vi "范围内渐变-颜色.vi"() -> ()   [LabVIEW 2013]
panel:
  in  "呼吸间隔ms":u32=250
  in  "刷新频率ms":u32=20
  out "波形图表":dbl(graph)
  out "Color":u32(colorbox) caption="颜色"
  in  "B动态范围":u8(slide) scale=1.0..50.0
  in  "R常量":u8(slide) scale=0.0..255.0
  in  "停止按钮":bool
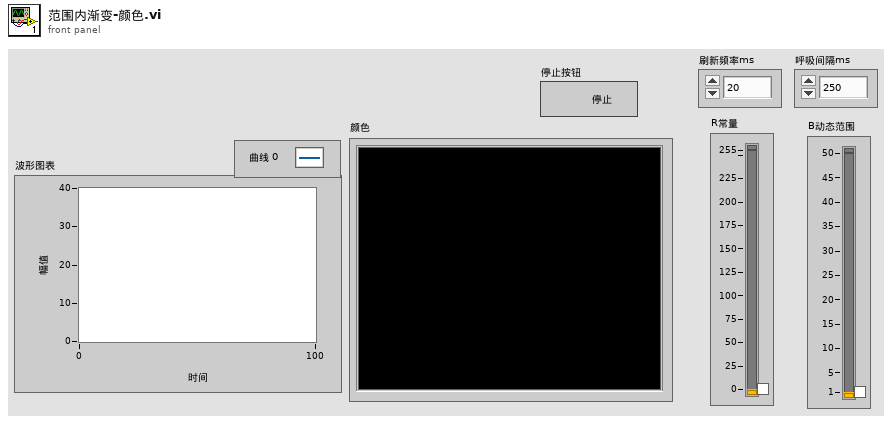
[diagram p1: front panel]
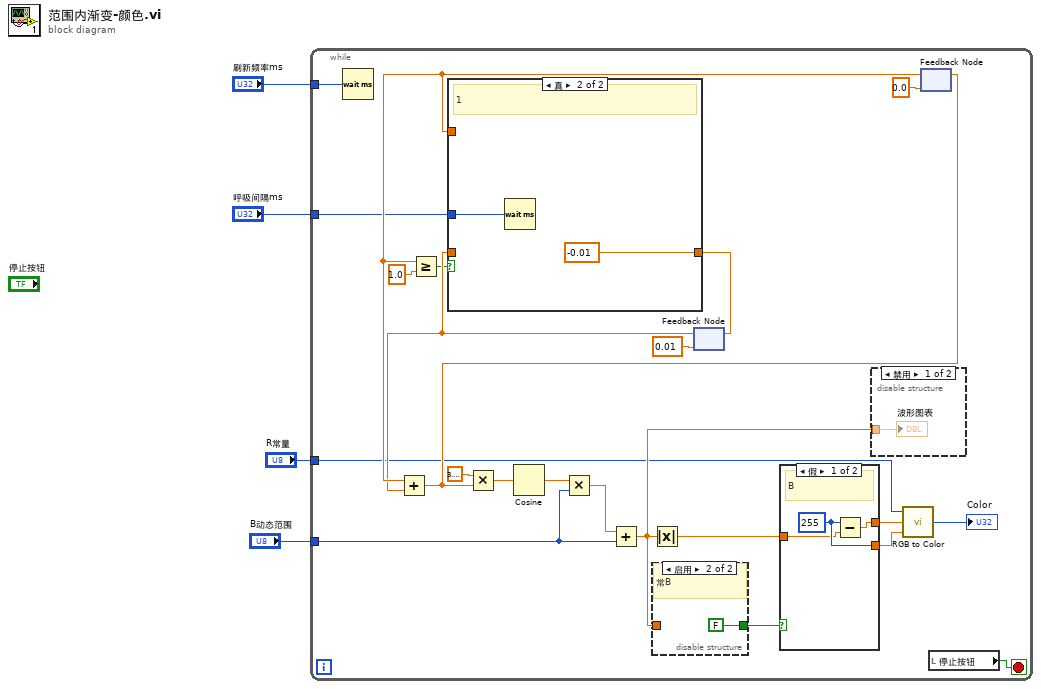
[diagram p0: block diagram]
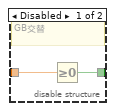
[diagram p3: hidden frame]
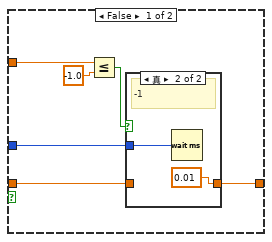
[diagram p4: hidden frame]
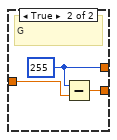
[diagram p6: hidden frame]
diagram:
  n1 = while {
    tunnel: "刷新频率ms" -> [w8]
    tunnel: "呼吸间隔ms" -> [w7]
    tunnel: "B动态范围" -> [w6]
    tunnel: "R常量" -> [w5]
    stop <- w22 stop-if-true
    n2 = Wait (ms)(milliseconds to wait=w8) -> ()  [unwired: 1 out]
    n3 = feedback #1(0.01 ("y")) -> (w13:dbl)
    n4 = feedback #2(0.0 ("y")) -> (w15:dbl)
    n5 = Add(x=w15, y=w13) -> (x+y=w18:dbl)
    n6 = Greater Or Equal?(x=w15, y=1.0) -> (x >= y?=w10:bool)
    n7 = case shown="真" w10 {
      tunnel: [w34 -0.01 ("y")] -> w12
      tunnel: w15 -> [w37 _]
      tunnel: w13 -> [w35 _]
      tunnel: w7 -> [w32 w41]
      frame False {
        n8 = Less Or Equal?(x=w37, y=-1.0) -> (x <= y?=w33:bool)
        n9 = case shown="真" w33 {
          tunnel: w35 -> [w38 _]
          tunnel: [w38 0.01 ("y")] -> w34
          tunnel: w32 -> [_ w39]
          frame False {
          }
          frame True {
            # "-1"
            n10 = Wait (ms)(milliseconds to wait=w39) -> ()  [unwired: 1 out]
          }
        }
      }
      frame True {
        # "1"
        n11 = Wait (ms)(milliseconds to wait=w41) -> ()  [unwired: 1 out]
      }
    }
    n12 = Multiply(x=3.141592653589793, y=w18) -> (x*y=w20:dbl)
    n13 = Cosine(x=w20) -> (cos(x)=w21:dbl)
    n14 = Multiply(x=w21, y=w6) -> (x*y=w11:dbl)
    n15 = Add(x=w11, y=w6) -> (x+y=w9:dbl)
    n16 = Absolute Value(x=w9) -> (abs(x)=w23:dbl)
    n17 = disable-structure shown="启用" {
      disable-tunnel: [w30 FALSE] -> w26
      disable-tunnel: w9 -> [w29 _]
      frame Disabled {
        # "GB交替"
        n18 = Greater Or Equal To 0?(x=w29) -> (x >= 0?=w30:bool)
      }
      frame Enabled {
        # "常B"
      }
    }
    n19 = feedback-in #1(w12) -> ()
    n20 = case shown="假" w26 {
      tunnel: w23 -> [w44 w48]
      tunnel: [w45 w47] -> w25
      tunnel: [w43 w46] -> w24
      frame False {
        w45 = u8 255 ("G")
        # "B"
        n21 = Subtract(x=w45, y=w44) -> (x-y=w43:dbl)
      }
      frame True {
        w46 = u8 255 ("G")
        # "G"
        n22 = Subtract(x=w46, y=w48) -> (x-y=w47:dbl)
      }
    }
    n23 = disable-structure shown="禁用" {
      disable-tunnel: w9 -> [w28 _]
      frame Disabled {
        "波形图表" <- w28
      }
      frame Enabled {
      }
    }
    n24 = call <vilib>:"RGB to Color.vi"("B"=w25, "G"=w24, "R"=w5) -> ("Color"=→"Color":u32)
    n25 = feedback-in #2(w18) -> ()
    n26 = local read "停止按钮"() -> (w22:bool)
  }
